vi "Server Op Num.vi"(11 "Server Op Num":i32) -> (2 "error out":errorcluster, 3 "Server Operation":T1)   [LabVIEW 2020, in "obs-websocket.lvlib"]
uses:
  obs-websocket.lvlib
  Server Operation.ctl
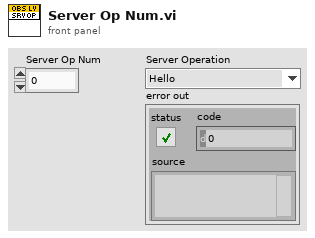
[diagram p1: front panel]
types:
  T1 = typedef "obs-websocket.lvlib/Server Operation.ctl" = enum16{"Hello", "Identified", "Event", "RequestResponse", "RequestBatchResponse"}
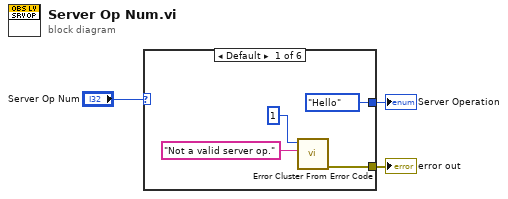
[diagram p0: block diagram]
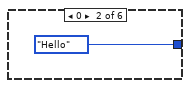
[diagram p2: hidden frame]
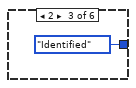
[diagram p3: hidden frame]
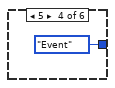
[diagram p4: hidden frame]
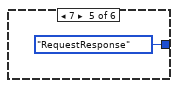
[diagram p5: hidden frame]
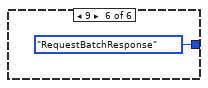
[diagram p6: hidden frame]
diagram:
  n1 = case shown="Default" "Server Op Num" {
    tunnel: [Server_Operation."Hello" ("Server Operation") Server_Operation."Hello" ("Server Operation") Server_Operation."Identified" ("Server Operation") Server_Operation."Event" ("Server Operation") Server_Operation."RequestResponse" ("Server Operation") Server_Operation."RequestBatchResponse" ("Server Operation")] -> w2
    tunnel: [w4 _ _ _ _ _] -> w1
    frame Default {
      n2 = call <vilib>:"Error Cluster From Error Code.vi"("error message (\"\")"="Not a valid server op." ("error message (\"\")"), "error code (0)"=1) -> ("error out"=w4:errorcluster)  [unwired: 7 in]
    }
    frame 0 {
    }
    frame 2 {
    }
    frame 5 {
    }
    frame 7 {
    }
    frame 9 {
    }
  }
  "Server Operation" <- w2
  "error out" <- w1
